vi "例4_IO.vi"() -> ()   [LabVIEW 2012]
panel:
  in  "EtherCAT  IO输出数":dbl
  in  "软件复位":bool
  in  "硬件复位":bool
  in  "总线状态":string
  in  "退出程序":bool
  in  "卡号":dbl
  in  "EtherCAT  IO输入数":dbl
  in  "15":bool
  in  "14":bool
  in  "7":bool
  in  "6":bool
  in  "13":bool
  in  "12":bool
  in  "11":bool
  in  "10":bool
  in  "9":bool
  in  "8":bool
  in  "5":bool
  in  "4":bool
  in  "3":bool
  in  "2":bool
  in  "1":bool
  in  "0":bool
  out "15":bool
  out "14":bool
  out "7":bool
  out "6":bool
  out "13":bool
  out "12":bool
  out "11":bool
  out "10":bool
  out "9":bool
  out "8":bool
  out "5":bool
  out "4":bool
  out "3":bool
  out "2":bool
  out "1":bool
  out "0":bool
  in  "7":bool
  in  "6":bool
  in  "5":bool
  in  "4":bool
  in  "3":bool
  in  "2":bool
  in  "1":bool
  in  "0":bool
  out "7":bool
  out "6":bool
  out "5":bool
  out "4":bool
  out "3":bool
  out "2":bool
  out "1":bool
  out "0":bool
  # "通用输入口（0~7）"
  # "EtherCAT  IO"
  # "通用输出口（0~7）"
  # "EtherCAT-输入口（0~15）"
  # "复位操作及总线状态"
  # "EtherCAT-输出口（0~15）"
  # "注：本例程位DMC—E3032总线卡接了一个EM32DX—E1EtherCAT总线IO扩展模块（16入16出）"
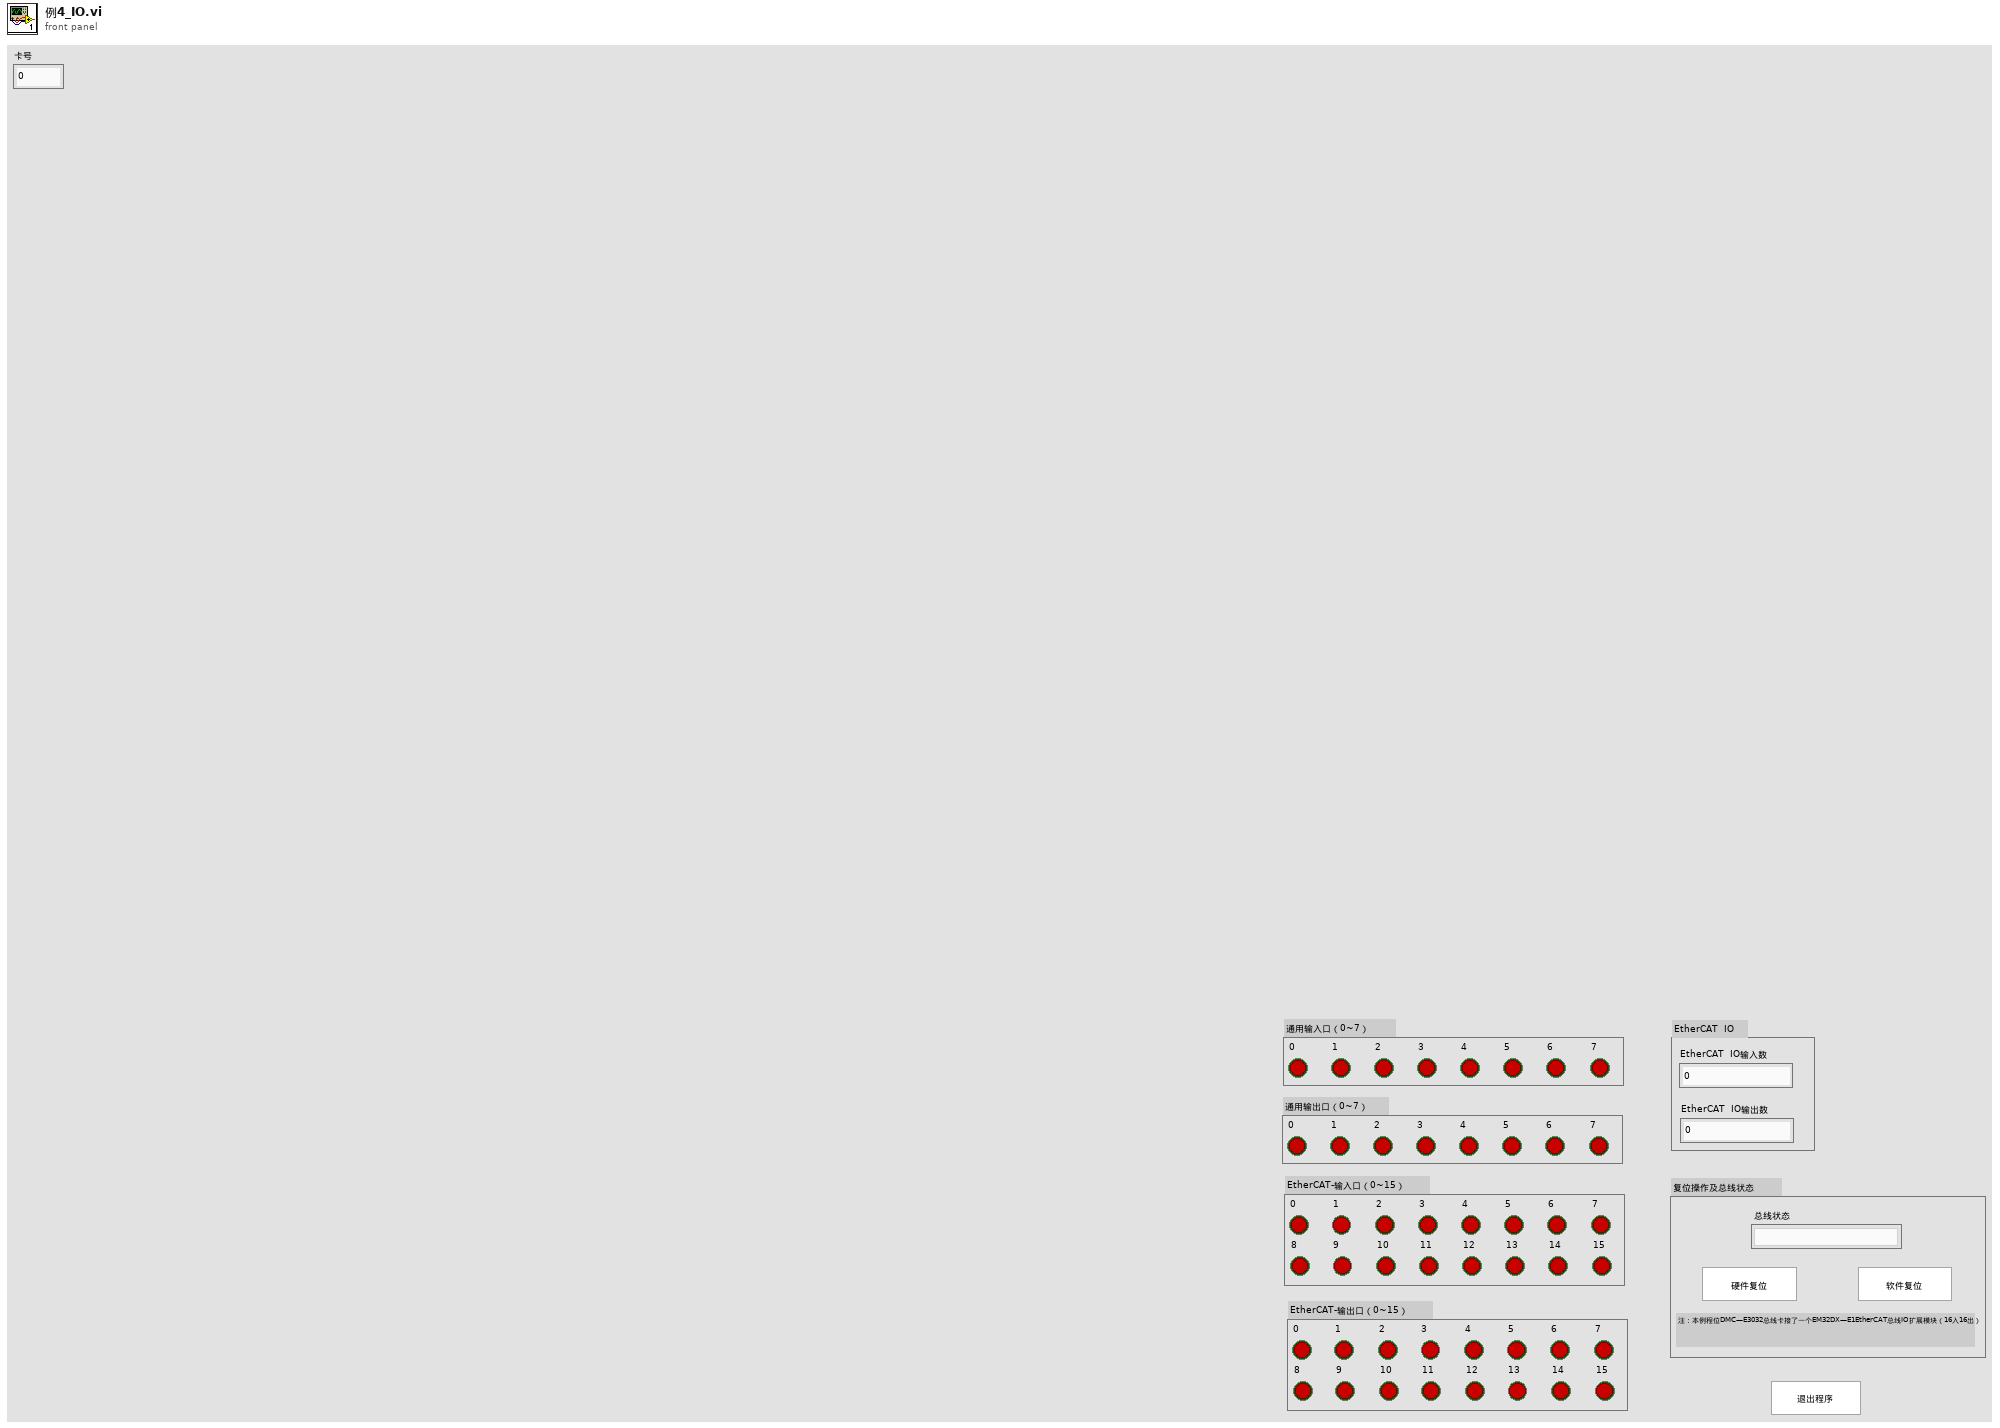
[diagram p1: front panel]
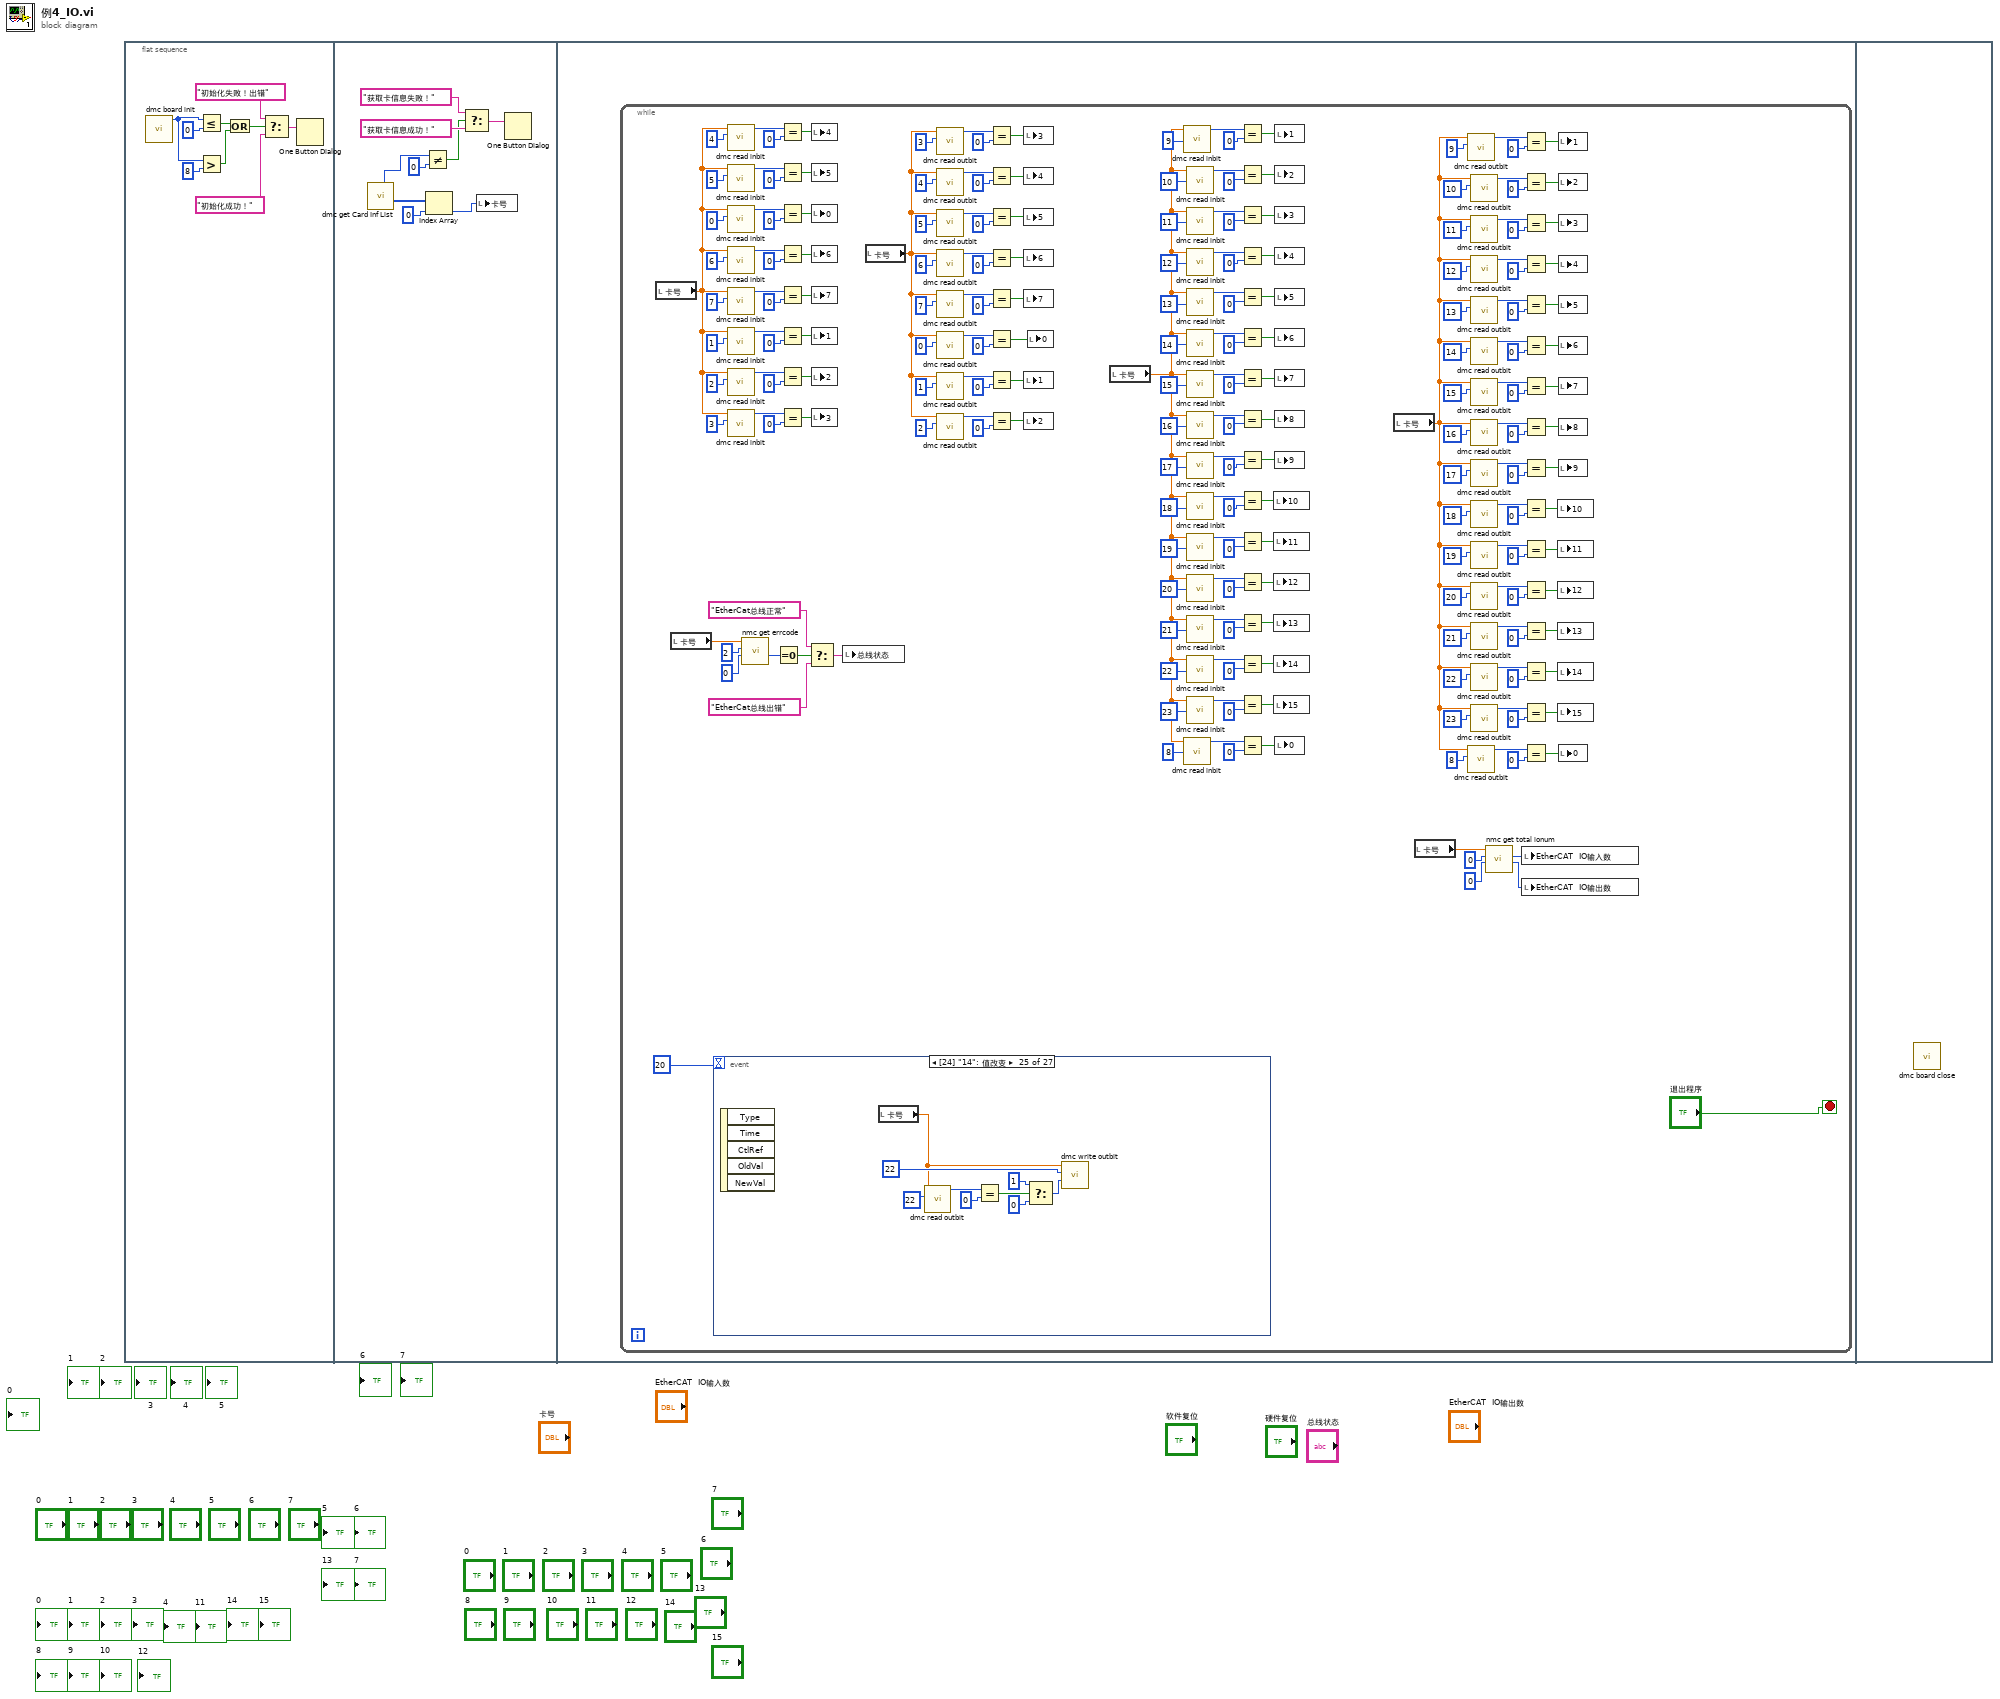
[diagram p0: block diagram]
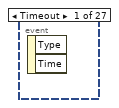
[diagram p2: hidden frame]
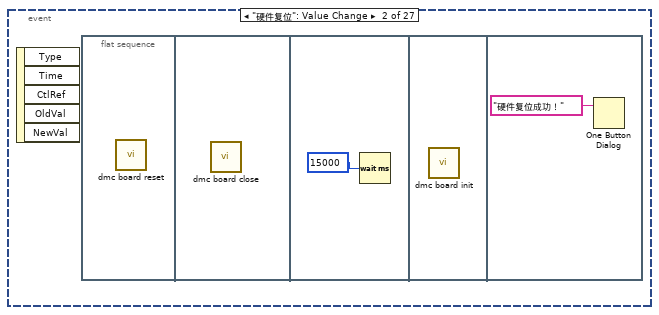
[diagram p3: hidden frame]
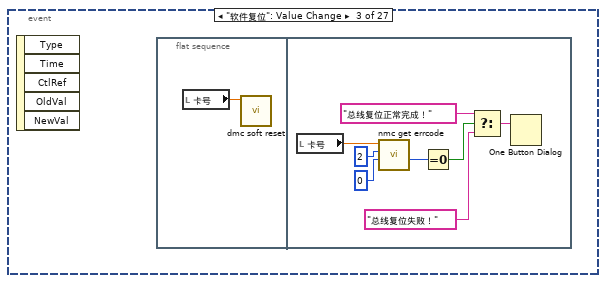
[diagram p4: hidden frame]
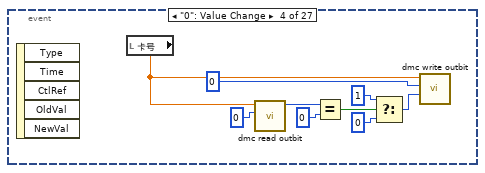
[diagram p5: hidden frame]
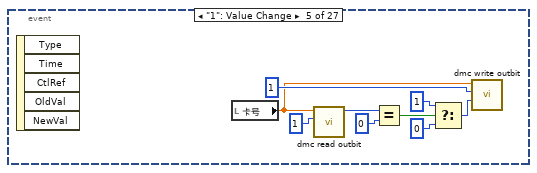
[diagram p6: hidden frame]
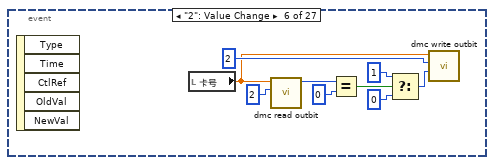
[diagram p7: hidden frame]
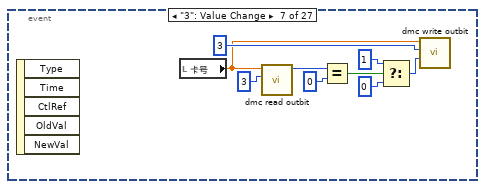
[diagram p8: hidden frame]
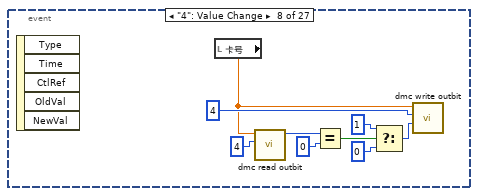
[diagram p9: hidden frame]
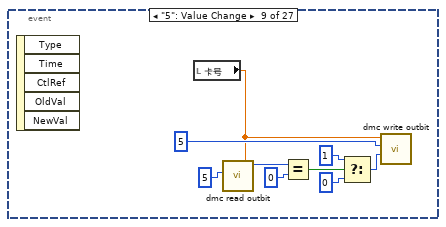
[diagram p10: hidden frame]
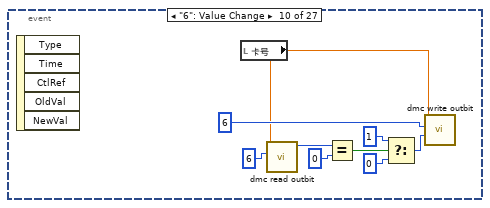
[diagram p11: hidden frame]
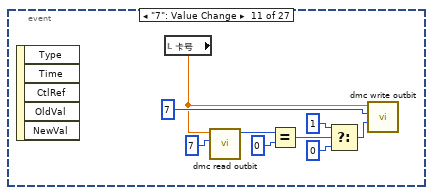
[diagram p12: hidden frame]
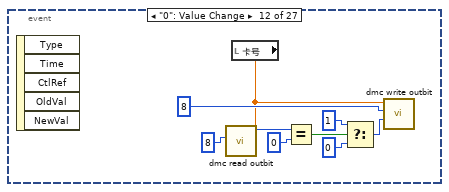
[diagram p13: hidden frame]
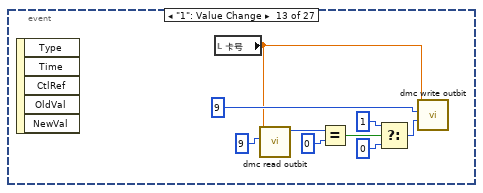
[diagram p14: hidden frame]
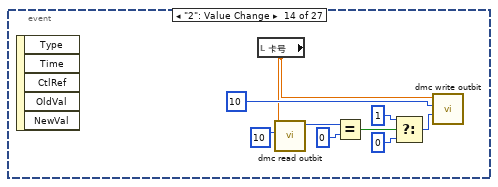
[diagram p15: hidden frame]
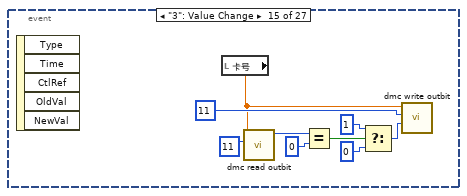
[diagram p16: hidden frame]
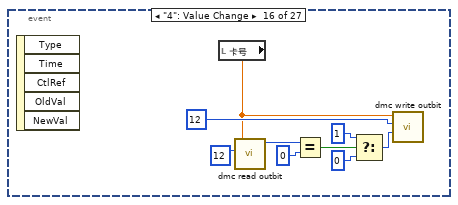
[diagram p17: hidden frame]
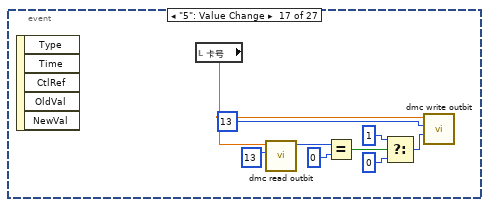
[diagram p18: hidden frame]
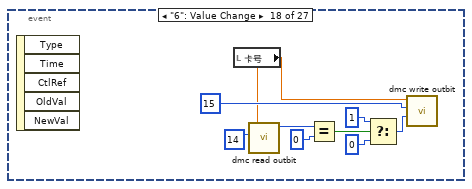
[diagram p19: hidden frame]
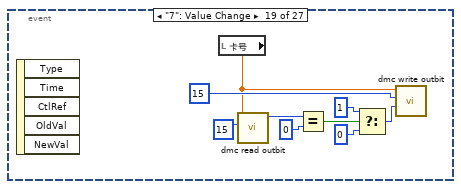
[diagram p20: hidden frame]
diagram:
  n1 = flat-sequence {
    frame #0 {
      n2 = call "dmc board init.vi"() -> ("function return"=w2:i16)  [unwired: 10 in, 1 out]
      n3 = Less Or Equal?(x=w2, y=0) -> (x <= y?=w5:bool)
      n4 = Greater?(x=w2, y=8) -> (0:w4:bool)
      n5 = Or(x=w5, y=w4) -> (x .or. y?=w6:bool)
      n6 = Select(t="初始化失败！出错", s=w6, f="初始化成功！") -> (s? t:f=w8:string)
      n7 = One Button Dialog(message=w8) -> ()  [unwired: 1 in, 1 out]
    }
    frame #1 {
      n8 = call "dmc get Card Inf List.vi"() -> ("CardIdList out"=w12:u16[], "function return"=w13:i16)  [unwired: 7 in, 3 out]
      n9 = Not Equal?(x=w13, y=0) -> (x != y?=w15:bool)
      n10 = Index Array(array=w12, index=0) -> (element=w10:u16)
      n11 = Select(t="获取卡信息失败！", s=w15, f="获取卡信息成功！") -> (s? t:f=w18:string)
      n12 = local write "卡号"(w10) -> ()
      n13 = One Button Dialog(message=w18) -> ()  [unwired: 1 in, 1 out]
    }
    frame #2 {
      n14 = while {
        stop <- "退出程序" stop-if-true
        n15 = local read "卡号"() -> (w197:dbl)
        n16 = local read "卡号"() -> (w19:dbl)
        n17 = event shown="[24] \"14\": 值改变" {
          selector: _ -> [_ _ _ _ _ _ _ _ _ _ _ _ _ _ _ _ _ _ _ _ _ _ _ _ _ _ _]
          dyn-events: _ -> [_ _ _ _ _ _ _ _ _ _ _ _ _ _ _ _ _ _ _ _ _ _ _ _ _ _ _]
          timeout: 20 -> [_ _ _ _ _ _ _ _ _ _ _ _ _ _ _ _ _ _ _ _ _ _ _ _ _ _ _]
          event Timeout {
            n18 = event-data() -> ()  [unwired: 1 in, 2 out]
          }
          event "硬件复位": Value Change {
            n19 = event-data() -> ()  [unwired: 1 in, 5 out]
            n20 = flat-sequence {
              frame #0 {
                n21 = call "dmc board reset.vi"() -> ()  [unwired: 10 in, 2 out]
              }
              frame #1 {
                n22 = call "dmc board close.vi"() -> ()  [unwired: 10 in, 2 out]
              }
              frame #2 {
                n23 = Wait (ms)(milliseconds to wait=15000) -> ()  [unwired: 1 out]
              }
              frame #3 {
                n24 = call "dmc board init.vi"() -> ()  [unwired: 10 in, 2 out]
              }
              frame #4 {
                n25 = One Button Dialog(message="硬件复位成功！") -> ()  [unwired: 1 in, 1 out]
              }
            }
          }
          event "软件复位": Value Change {
            n26 = event-data() -> ()  [unwired: 1 in, 5 out]
            n27 = flat-sequence {
              frame #0 {
                n28 = local read "卡号"() -> (w232:dbl)
                n29 = call "dmc soft reset.vi"("CardNo"=w232) -> ()  [unwired: 9 in, 2 out]
              }
              frame #1 {
                n30 = local read "卡号"() -> (w233:dbl)
                n31 = call "nmc get errcode.vi"("Errcode"=0, "channel"=2, "CardNo"=w233) -> ("Errcode out"=w237:u16)  [unwired: 6 in, 2 out]
                n32 = Equal To 0?(x=w237) -> (x = 0?=w238:bool)
                n33 = Select(t="总线复位正常完成！" ("当前状态"), s=w238, f="总线复位失败！" ("当前状态")) -> (s? t:f=w234:string)
                n34 = One Button Dialog(message=w234) -> ()  [unwired: 1 in, 1 out]
              }
            }
          }
          event "0": Value Change {
            n35 = event-data() -> ()  [unwired: 1 in, 5 out]
            n36 = local read "卡号"() -> (w241:dbl)
            n37 = call "dmc read outbit.vi"("bitno"=0, "CardNo"=w241) -> ("function return"=w248:i16)  [unwired: 8 in, 1 out]
            n38 = Equal?(x=w248, y=0) -> (x = y?=w246:bool)
            n39 = Select(t=1, s=w246, f=0) -> (s? t:f=w242:i32)
            n40 = call "dmc write outbit.vi"("on_off"=w242, "bitno"=0, "CardNo"=w241) -> ()  [unwired: 7 in, 2 out]
          }
          event "1": Value Change {
            n41 = event-data() -> ()  [unwired: 1 in, 5 out]
            n42 = local read "卡号"() -> (w250:dbl)
            n43 = call "dmc read outbit.vi"("bitno"=1, "CardNo"=w250) -> ("function return"=w257:i16)  [unwired: 8 in, 1 out]
            n44 = Equal?(x=w257, y=0) -> (x = y?=w255:bool)
            n45 = Select(t=1, s=w255, f=0) -> (s? t:f=w251:i32)
            n46 = call "dmc write outbit.vi"("on_off"=w251, "bitno"=1, "CardNo"=w250) -> ()  [unwired: 7 in, 2 out]
          }
          event "2": Value Change {
            n47 = event-data() -> ()  [unwired: 1 in, 5 out]
            n48 = local read "卡号"() -> (w259:dbl)
            n49 = call "dmc read outbit.vi"("bitno"=2, "CardNo"=w259) -> ("function return"=w266:i16)  [unwired: 8 in, 1 out]
            n50 = Equal?(x=w266, y=0) -> (x = y?=w264:bool)
            n51 = Select(t=1, s=w264, f=0) -> (s? t:f=w260:i32)
            n52 = call "dmc write outbit.vi"("on_off"=w260, "bitno"=2, "CardNo"=w259) -> ()  [unwired: 7 in, 2 out]
          }
          event "3": Value Change {
            n53 = event-data() -> ()  [unwired: 1 in, 5 out]
            n54 = local read "卡号"() -> (w268:dbl)
            n55 = call "dmc read outbit.vi"("bitno"=3, "CardNo"=w268) -> ("function return"=w275:i16)  [unwired: 8 in, 1 out]
            n56 = Equal?(x=w275, y=0) -> (x = y?=w273:bool)
            n57 = Select(t=1, s=w273, f=0) -> (s? t:f=w269:i32)
            n58 = call "dmc write outbit.vi"("on_off"=w269, "bitno"=3, "CardNo"=w268) -> ()  [unwired: 7 in, 2 out]
          }
          event "4": Value Change {
            n59 = event-data() -> ()  [unwired: 1 in, 5 out]
            n60 = local read "卡号"() -> (w277:dbl)
            n61 = call "dmc read outbit.vi"("bitno"=4, "CardNo"=w277) -> ("function return"=w284:i16)  [unwired: 8 in, 1 out]
            n62 = Equal?(x=w284, y=0) -> (x = y?=w282:bool)
            n63 = Select(t=1, s=w282, f=0) -> (s? t:f=w278:i32)
            n64 = call "dmc write outbit.vi"("on_off"=w278, "bitno"=4, "CardNo"=w277) -> ()  [unwired: 7 in, 2 out]
          }
          event "5": Value Change {
            n65 = event-data() -> ()  [unwired: 1 in, 5 out]
            n66 = local read "卡号"() -> (w286:dbl)
            n67 = call "dmc read outbit.vi"("bitno"=5, "CardNo"=w286) -> ("function return"=w288:i16)  [unwired: 8 in, 1 out]
            n68 = Equal?(x=w288, y=0) -> (x = y?=w290:bool)
            n69 = Select(t=1, s=w290, f=0) -> (s? t:f=w294:i32)
            n70 = call "dmc write outbit.vi"("on_off"=w294, "bitno"=5, "CardNo"=w286) -> ()  [unwired: 7 in, 2 out]
          }
          event "6": Value Change {
            n71 = event-data() -> ()  [unwired: 1 in, 5 out]
            n72 = local read "卡号"() -> (w295:dbl)
            n73 = call "dmc read outbit.vi"("bitno"=6, "CardNo"=w295) -> ("function return"=w302:i16)  [unwired: 8 in, 1 out]
            n74 = Equal?(x=w302, y=0) -> (x = y?=w300:bool)
            n75 = Select(t=1, s=w300, f=0) -> (s? t:f=w296:i32)
            n76 = call "dmc write outbit.vi"("on_off"=w296, "bitno"=6, "CardNo"=w295) -> ()  [unwired: 7 in, 2 out]
          }
          event "7": Value Change {
            n77 = event-data() -> ()  [unwired: 1 in, 5 out]
            n78 = local read "卡号"() -> (w304:dbl)
            n79 = call "dmc read outbit.vi"("bitno"=7, "CardNo"=w304) -> ("function return"=w311:i16)  [unwired: 8 in, 1 out]
            n80 = Equal?(x=w311, y=0) -> (x = y?=w309:bool)
            n81 = Select(t=1, s=w309, f=0) -> (s? t:f=w305:i32)
            n82 = call "dmc write outbit.vi"("on_off"=w305, "bitno"=7, "CardNo"=w304) -> ()  [unwired: 7 in, 2 out]
          }
          event "0": Value Change {
            n83 = event-data() -> ()  [unwired: 1 in, 5 out]
            n84 = local read "卡号"() -> (w313:dbl)
            n85 = call "dmc read outbit.vi"("bitno"=8, "CardNo"=w313) -> ("function return"=w320:i16)  [unwired: 8 in, 1 out]
            n86 = Equal?(x=w320, y=0) -> (x = y?=w318:bool)
            n87 = Select(t=1, s=w318, f=0) -> (s? t:f=w314:i32)
            n88 = call "dmc write outbit.vi"("on_off"=w314, "bitno"=8, "CardNo"=w313) -> ()  [unwired: 7 in, 2 out]
          }
          event "1": Value Change {
            n89 = event-data() -> ()  [unwired: 1 in, 5 out]
            n90 = local read "卡号"() -> (w322:dbl)
            n91 = call "dmc read outbit.vi"("bitno"=9, "CardNo"=w322) -> ("function return"=w329:i16)  [unwired: 8 in, 1 out]
            n92 = Equal?(x=w329, y=0) -> (x = y?=w327:bool)
            n93 = Select(t=1, s=w327, f=0) -> (s? t:f=w323:i32)
            n94 = call "dmc write outbit.vi"("on_off"=w323, "bitno"=9, "CardNo"=w322) -> ()  [unwired: 7 in, 2 out]
          }
          event "2": Value Change {
            n95 = event-data() -> ()  [unwired: 1 in, 5 out]
            n96 = local read "卡号"() -> (w331:dbl)
            n97 = call "dmc read outbit.vi"("bitno"=10, "CardNo"=w331) -> ("function return"=w338:i16)  [unwired: 8 in, 1 out]
            n98 = Equal?(x=w338, y=0) -> (x = y?=w336:bool)
            n99 = Select(t=1, s=w336, f=0) -> (s? t:f=w332:i32)
            n100 = call "dmc write outbit.vi"("on_off"=w332, "bitno"=10, "CardNo"=w331) -> ()  [unwired: 7 in, 2 out]
          }
          event "3": Value Change {
            n101 = event-data() -> ()  [unwired: 1 in, 5 out]
            n102 = local read "卡号"() -> (w340:dbl)
            n103 = call "dmc read outbit.vi"("bitno"=11, "CardNo"=w340) -> ("function return"=w347:i16)  [unwired: 8 in, 1 out]
            n104 = Equal?(x=w347, y=0) -> (x = y?=w345:bool)
            n105 = Select(t=1, s=w345, f=0) -> (s? t:f=w341:i32)
            n106 = call "dmc write outbit.vi"("on_off"=w341, "bitno"=11, "CardNo"=w340) -> ()  [unwired: 7 in, 2 out]
          }
          event "4": Value Change {
            n107 = event-data() -> ()  [unwired: 1 in, 5 out]
            n108 = local read "卡号"() -> (w349:dbl)
            n109 = call "dmc read outbit.vi"("bitno"=12, "CardNo"=w349) -> ("function return"=w356:i16)  [unwired: 8 in, 1 out]
            n110 = Equal?(x=w356, y=0) -> (x = y?=w354:bool)
            n111 = Select(t=1, s=w354, f=0) -> (s? t:f=w350:i32)
            n112 = call "dmc write outbit.vi"("on_off"=w350, "bitno"=12, "CardNo"=w349) -> ()  [unwired: 7 in, 2 out]
          }
          event "5": Value Change {
            n113 = event-data() -> ()  [unwired: 1 in, 5 out]
            n114 = local read "卡号"() -> (w358:dbl)
            n115 = call "dmc read outbit.vi"("bitno"=13, "CardNo"=w358) -> ("function return"=w360:i16)  [unwired: 8 in, 1 out]
            n116 = Equal?(x=w360, y=0) -> (x = y?=w362:bool)
            n117 = Select(t=1, s=w362, f=0) -> (s? t:f=w366:i32)
            n118 = call "dmc write outbit.vi"("on_off"=w366, "bitno"=13, "CardNo"=w358) -> ()  [unwired: 7 in, 2 out]
          }
          event "6": Value Change {
            n119 = event-data() -> ()  [unwired: 1 in, 5 out]
            n120 = local read "卡号"() -> (w367:dbl)
            n121 = call "dmc read outbit.vi"("bitno"=14, "CardNo"=w367) -> ("function return"=w374:i16)  [unwired: 8 in, 1 out]
            n122 = Equal?(x=w374, y=0) -> (x = y?=w372:bool)
            n123 = Select(t=1, s=w372, f=0) -> (s? t:f=w368:i32)
            n124 = call "dmc write outbit.vi"("on_off"=w368, "bitno"=15, "CardNo"=w367) -> ()  [unwired: 7 in, 2 out]
          }
          event "7": Value Change {
            n125 = event-data() -> ()  [unwired: 1 in, 5 out]
            n126 = local read "卡号"() -> (w376:dbl)
            n127 = call "dmc read outbit.vi"("bitno"=15, "CardNo"=w376) -> ("function return"=w383:i16)  [unwired: 8 in, 1 out]
            n128 = Equal?(x=w383, y=0) -> (x = y?=w381:bool)
            n129 = Select(t=1, s=w381, f=0) -> (s? t:f=w377:i32)
            n130 = call "dmc write outbit.vi"("on_off"=w377, "bitno"=15, "CardNo"=w376) -> ()  [unwired: 7 in, 2 out]
          }
          event "8": Value Change {
            n131 = event-data() -> ()  [unwired: 1 in, 5 out]
            n132 = local read "卡号"() -> (w385:dbl)
            n133 = call "dmc read outbit.vi"("bitno"=16, "CardNo"=w385) -> ("function return"=w392:i16)  [unwired: 8 in, 1 out]
            n134 = Equal?(x=w392, y=0) -> (x = y?=w390:bool)
            n135 = Select(t=1, s=w390, f=0) -> (s? t:f=w386:i32)
            n136 = call "dmc write outbit.vi"("on_off"=w386, "bitno"=16, "CardNo"=w385) -> ()  [unwired: 7 in, 2 out]
          }
          event "9": Value Change {
            n137 = event-data() -> ()  [unwired: 1 in, 5 out]
            n138 = local read "卡号"() -> (w394:dbl)
            n139 = call "dmc read outbit.vi"("bitno"=17, "CardNo"=w394) -> ("function return"=w396:i16)  [unwired: 8 in, 1 out]
            n140 = Equal?(x=w396, y=0) -> (x = y?=w398:bool)
            n141 = Select(t=1, s=w398, f=0) -> (s? t:f=w402:i32)
            n142 = call "dmc write outbit.vi"("on_off"=w402, "bitno"=17, "CardNo"=w394) -> ()  [unwired: 7 in, 2 out]
          }
          event "10": Value Change {
            n143 = event-data() -> ()  [unwired: 1 in, 5 out]
            n144 = local read "卡号"() -> (w403:dbl)
            n145 = call "dmc read outbit.vi"("bitno"=18, "CardNo"=w403) -> ("function return"=w410:i16)  [unwired: 8 in, 1 out]
            n146 = Equal?(x=w410, y=0) -> (x = y?=w408:bool)
            n147 = Select(t=1, s=w408, f=0) -> (s? t:f=w404:i32)
            n148 = call "dmc write outbit.vi"("on_off"=w404, "bitno"=18, "CardNo"=w403) -> ()  [unwired: 7 in, 2 out]
          }
          event "12": Value Change {
            n149 = event-data() -> ()  [unwired: 1 in, 5 out]
            n150 = local read "卡号"() -> (w412:dbl)
            n151 = call "dmc read outbit.vi"("bitno"=20, "CardNo"=w412) -> ("function return"=w419:i16)  [unwired: 8 in, 1 out]
            n152 = Equal?(x=w419, y=0) -> (x = y?=w417:bool)
            n153 = Select(t=1, s=w417, f=0) -> (s? t:f=w413:i32)
            n154 = call "dmc write outbit.vi"("on_off"=w413, "bitno"=20, "CardNo"=w412) -> ()  [unwired: 7 in, 2 out]
          }
          event "13": Value Change {
            n155 = event-data() -> ()  [unwired: 1 in, 5 out]
            n156 = local read "卡号"() -> (w421:dbl)
            n157 = call "dmc read outbit.vi"("bitno"=21, "CardNo"=w421) -> ("function return"=w428:i16)  [unwired: 8 in, 1 out]
            n158 = Equal?(x=w428, y=0) -> (x = y?=w426:bool)
            n159 = Select(t=1, s=w426, f=0) -> (s? t:f=w422:i32)
            n160 = call "dmc write outbit.vi"("on_off"=w422, "bitno"=21, "CardNo"=w421) -> ()  [unwired: 7 in, 2 out]
          }
          event "14": Value Change {
            n161 = event-data() -> ()  [unwired: 1 in, 5 out]
            n162 = local read "卡号"() -> (w430:dbl)
            n163 = call "dmc read outbit.vi"("bitno"=22, "CardNo"=w430) -> ("function return"=w437:i16)  [unwired: 8 in, 1 out]
            n164 = Equal?(x=w437, y=0) -> (x = y?=w435:bool)
            n165 = Select(t=1, s=w435, f=0) -> (s? t:f=w431:i32)
            n166 = call "dmc write outbit.vi"("on_off"=w431, "bitno"=22, "CardNo"=w430) -> ()  [unwired: 7 in, 2 out]
          }
          event "15": Value Change {
            n167 = event-data() -> ()  [unwired: 1 in, 5 out]
            n168 = local read "卡号"() -> (w439:dbl)
            n169 = call "dmc read outbit.vi"("bitno"=23, "CardNo"=w439) -> ("function return"=w446:i16)  [unwired: 8 in, 1 out]
            n170 = Equal?(x=w446, y=0) -> (x = y?=w444:bool)
            n171 = Select(t=1, s=w444, f=0) -> (s? t:f=w440:i32)
            n172 = call "dmc write outbit.vi"("on_off"=w440, "bitno"=23, "CardNo"=w439) -> ()  [unwired: 7 in, 2 out]
          }
          event "11": Value Change {
            n173 = event-data() -> ()  [unwired: 1 in, 5 out]
            n174 = local read "卡号"() -> (w448:dbl)
            n175 = call "dmc read outbit.vi"("bitno"=19, "CardNo"=w448) -> ("function return"=w455:i16)  [unwired: 8 in, 1 out]
            n176 = Equal?(x=w455, y=0) -> (x = y?=w453:bool)
            n177 = Select(t=1, s=w453, f=0) -> (s? t:f=w449:i32)
            n178 = call "dmc write outbit.vi"("on_off"=w449, "bitno"=19, "CardNo"=w448) -> ()  [unwired: 7 in, 2 out]
          }
        }
        n179 = call "dmc read inbit.vi"("bitno"=4, "CardNo"=w197) -> ("function return"=w211:i16)  [unwired: 8 in, 1 out]
        n180 = call "dmc read inbit.vi"("bitno"=5, "CardNo"=w197) -> ("function return"=w207:i16)  [unwired: 8 in, 1 out]
        n181 = call "dmc read inbit.vi"("bitno"=0, "CardNo"=w197) -> ("function return"=w228:i16)  [unwired: 8 in, 1 out]
        n182 = call "dmc read inbit.vi"("bitno"=6, "CardNo"=w197) -> ("function return"=w203:i16)  [unwired: 8 in, 1 out]
        n183 = call "dmc read inbit.vi"("bitno"=7, "CardNo"=w197) -> ("function return"=w200:i16)  [unwired: 8 in, 1 out]
        n184 = call "dmc read inbit.vi"("bitno"=1, "CardNo"=w197) -> ("function return"=w222:i16)  [unwired: 8 in, 1 out]
        n185 = call "dmc read inbit.vi"("bitno"=2, "CardNo"=w197) -> ("function return"=w218:i16)  [unwired: 8 in, 1 out]
        n186 = call "dmc read inbit.vi"("bitno"=3, "CardNo"=w197) -> ("function return"=w215:i16)  [unwired: 8 in, 1 out]
        n187 = call "nmc get errcode.vi"("Errcode"=0, "channel"=2, "CardNo"=w19) -> ("Errcode out"=w24:u16)  [unwired: 6 in, 2 out]
        n188 = Equal To 0?(x=w24) -> (x = 0?=w23:bool)
        n189 = Equal?(x=w211, y=0) -> (x = y?=w210:bool)
        n190 = Equal?(x=w207, y=0) -> (x = y?=w206:bool)
        n191 = Equal?(x=w228, y=0) -> (x = y?=w226:bool)
        n192 = Equal?(x=w203, y=0) -> (x = y?=w202:bool)
        n193 = Equal?(x=w200, y=0) -> (x = y?=w199:bool)
        n194 = Equal?(x=w222, y=0) -> (x = y?=w223:bool)
        n195 = Equal?(x=w218, y=0) -> (x = y?=w219:bool)
        n196 = Equal?(x=w215, y=0) -> (x = y?=w214:bool)
        n197 = Select(t="EtherCat总线正常" ("当前状态"), s=w23, f="EtherCat总线出错" ("当前状态")) -> (s? t:f=w20:string)
        n198 = local write "4"(w210) -> ()
        n199 = local write "5"(w206) -> ()
        n200 = local write "0"(w226) -> ()
        n201 = local write "6"(w202) -> ()
        n202 = local write "7"(w199) -> ()
        n203 = local write "1"(w223) -> ()
        n204 = local write "2"(w219) -> ()
        n205 = local write "3"(w214) -> ()
        n206 = local write "总线状态"(w20) -> ()
        n207 = local read "卡号"() -> (w164:dbl)
        n208 = call "dmc read outbit.vi"("bitno"=3, "CardNo"=w164) -> ("function return"=w184:i16)  [unwired: 8 in, 1 out]
        n209 = call "dmc read outbit.vi"("bitno"=4, "CardNo"=w164) -> ("function return"=w181:i16)  [unwired: 8 in, 1 out]
        n210 = call "dmc read outbit.vi"("bitno"=5, "CardNo"=w164) -> ("function return"=w178:i16)  [unwired: 8 in, 1 out]
        n211 = call "dmc read outbit.vi"("bitno"=6, "CardNo"=w164) -> ("function return"=w175:i16)  [unwired: 8 in, 1 out]
        n212 = call "dmc read outbit.vi"("bitno"=7, "CardNo"=w164) -> ("function return"=w172:i16)  [unwired: 8 in, 1 out]
        n213 = call "dmc read outbit.vi"("bitno"=0, "CardNo"=w164) -> ("function return"=w194:i16)  [unwired: 8 in, 1 out]
        n214 = call "dmc read outbit.vi"("bitno"=1, "CardNo"=w164) -> ("function return"=w190:i16)  [unwired: 8 in, 1 out]
        n215 = call "dmc read outbit.vi"("bitno"=2, "CardNo"=w164) -> ("function return"=w187:i16)  [unwired: 8 in, 1 out]
        n216 = Equal?(x=w184, y=0) -> (x = y?=w166:bool)
        n217 = Equal?(x=w181, y=0) -> (x = y?=w167:bool)
        n218 = Equal?(x=w178, y=0) -> (x = y?=w168:bool)
        n219 = Equal?(x=w175, y=0) -> (x = y?=w169:bool)
        n220 = Equal?(x=w172, y=0) -> (x = y?=w170:bool)
        n221 = Equal?(x=w194, y=0) -> (x = y?=w193:bool)
        n222 = Equal?(x=w190, y=0) -> (x = y?=w171:bool)
        n223 = Equal?(x=w187, y=0) -> (x = y?=w165:bool)
        n224 = local write "3"(w166) -> ()
        n225 = local write "4"(w167) -> ()
        n226 = local write "5"(w168) -> ()
        n227 = local write "6"(w169) -> ()
        n228 = local write "7"(w170) -> ()
        n229 = local write "1"(w171) -> ()
        n230 = local write "2"(w165) -> ()
        n231 = local write "0"(w193) -> ()
        n232 = local read "卡号"() -> (w115:dbl)
        n233 = call "dmc read inbit.vi"("bitno"=9, "CardNo"=w115) -> ("function return"=w157:i16)  [unwired: 8 in, 1 out]
        n234 = call "dmc read inbit.vi"("bitno"=8, "CardNo"=w115) -> ("function return"=w158:i16)  [unwired: 8 in, 1 out]
        n235 = call "dmc read inbit.vi"("bitno"=10, "CardNo"=w115) -> ("function return"=w161:i16)  [unwired: 8 in, 1 out]
        n236 = call "dmc read inbit.vi"("bitno"=11, "CardNo"=w115) -> ("function return"=w156:i16)  [unwired: 8 in, 1 out]
        n237 = call "dmc read inbit.vi"("bitno"=12, "CardNo"=w115) -> ("function return"=w155:i16)  [unwired: 8 in, 1 out]
        n238 = call "dmc read inbit.vi"("bitno"=13, "CardNo"=w115) -> ("function return"=w160:i16)  [unwired: 8 in, 1 out]
        n239 = call "dmc read inbit.vi"("bitno"=14, "CardNo"=w115) -> ("function return"=w109:i16)  [unwired: 8 in, 1 out]
        n240 = call "dmc read inbit.vi"("bitno"=15, "CardNo"=w115) -> ("function return"=w159:i16)  [unwired: 8 in, 1 out]
        n241 = call "dmc read inbit.vi"("bitno"=16, "CardNo"=w115) -> ("function return"=w151:i16)  [unwired: 8 in, 1 out]
        n242 = call "dmc read inbit.vi"("bitno"=17, "CardNo"=w115) -> ("function return"=w150:i16)  [unwired: 8 in, 1 out]
        n243 = call "dmc read inbit.vi"("bitno"=18, "CardNo"=w115) -> ("function return"=w114:i16)  [unwired: 8 in, 1 out]
        n244 = call "dmc read inbit.vi"("bitno"=19, "CardNo"=w115) -> ("function return"=w149:i16)  [unwired: 8 in, 1 out]
        n245 = call "dmc read inbit.vi"("bitno"=20, "CardNo"=w115) -> ("function return"=w148:i16)  [unwired: 8 in, 1 out]
        n246 = call "dmc read inbit.vi"("bitno"=21, "CardNo"=w115) -> ("function return"=w154:i16)  [unwired: 8 in, 1 out]
        n247 = call "dmc read inbit.vi"("bitno"=22, "CardNo"=w115) -> ("function return"=w153:i16)  [unwired: 8 in, 1 out]
        n248 = call "dmc read inbit.vi"("bitno"=23, "CardNo"=w115) -> ("function return"=w152:i16)  [unwired: 8 in, 1 out]
        n249 = Equal?(x=w157, y=0) -> (x = y?=w130:bool)
        n250 = Equal?(x=w161, y=0) -> (x = y?=w129:bool)
        n251 = Equal?(x=w156, y=0) -> (x = y?=w128:bool)
        n252 = Equal?(x=w155, y=0) -> (x = y?=w127:bool)
        n253 = Equal?(x=w160, y=0) -> (x = y?=w126:bool)
        n254 = Equal?(x=w109, y=0) -> (x = y?=w125:bool)
        n255 = Equal?(x=w159, y=0) -> (x = y?=w124:bool)
        n256 = Equal?(x=w151, y=0) -> (x = y?=w123:bool)
        n257 = Equal?(x=w150, y=0) -> (x = y?=w122:bool)
        n258 = Equal?(x=w114, y=0) -> (x = y?=w121:bool)
        n259 = Equal?(x=w149, y=0) -> (x = y?=w120:bool)
        n260 = Equal?(x=w148, y=0) -> (x = y?=w119:bool)
        n261 = Equal?(x=w154, y=0) -> (x = y?=w118:bool)
        n262 = Equal?(x=w153, y=0) -> (x = y?=w117:bool)
        n263 = Equal?(x=w152, y=0) -> (x = y?=w116:bool)
        n264 = Equal?(x=w158, y=0) -> (x = y?=w131:bool)
        n265 = local write "10"(w121) -> ()
        n266 = local write "11"(w120) -> ()
        n267 = local write "12"(w119) -> ()
        n268 = local write "13"(w118) -> ()
        n269 = local write "14"(w117) -> ()
        n270 = local write "15"(w116) -> ()
        n271 = local write "1"(w130) -> ()
        n272 = local write "2"(w129) -> ()
        n273 = local write "3"(w128) -> ()
        n274 = local write "4"(w127) -> ()
        n275 = local write "5"(w126) -> ()
        n276 = local write "6"(w125) -> ()
        n277 = local write "7"(w124) -> ()
        n278 = local write "8"(w123) -> ()
        n279 = local write "9"(w122) -> ()
        n280 = local write "0"(w131) -> ()
        n281 = local read "卡号"() -> (w48:dbl)
        n282 = local read "卡号"() -> (w31:dbl)
        n283 = call "dmc read outbit.vi"("bitno"=9, "CardNo"=w48) -> ("function return"=w89:i16)  [unwired: 8 in, 1 out]
        n284 = call "dmc read outbit.vi"("bitno"=8, "CardNo"=w48) -> ("function return"=w91:i16)  [unwired: 8 in, 1 out]
        n285 = call "dmc read outbit.vi"("bitno"=10, "CardNo"=w48) -> ("function return"=w87:i16)  [unwired: 8 in, 1 out]
        n286 = call "dmc read outbit.vi"("bitno"=11, "CardNo"=w48) -> ("function return"=w85:i16)  [unwired: 8 in, 1 out]
        n287 = call "dmc read outbit.vi"("bitno"=12, "CardNo"=w48) -> ("function return"=w83:i16)  [unwired: 8 in, 1 out]
        n288 = call "dmc read outbit.vi"("bitno"=13, "CardNo"=w48) -> ("function return"=w97:i16)  [unwired: 8 in, 1 out]
        n289 = call "dmc read outbit.vi"("bitno"=14, "CardNo"=w48) -> ("function return"=w95:i16)  [unwired: 8 in, 1 out]
        n290 = call "dmc read outbit.vi"("bitno"=15, "CardNo"=w48) -> ("function return"=w93:i16)  [unwired: 8 in, 1 out]
        n291 = call "dmc read outbit.vi"("bitno"=16, "CardNo"=w48) -> ("function return"=w75:i16)  [unwired: 8 in, 1 out]
        n292 = call "dmc read outbit.vi"("bitno"=17, "CardNo"=w48) -> ("function return"=w73:i16)  [unwired: 8 in, 1 out]
        n293 = call "dmc read outbit.vi"("bitno"=18, "CardNo"=w48) -> ("function return"=w71:i16)  [unwired: 8 in, 1 out]
        n294 = call "dmc read outbit.vi"("bitno"=19, "CardNo"=w48) -> ("function return"=w69:i16)  [unwired: 8 in, 1 out]
        n295 = call "dmc read outbit.vi"("bitno"=20, "CardNo"=w48) -> ("function return"=w67:i16)  [unwired: 8 in, 1 out]
        n296 = call "dmc read outbit.vi"("bitno"=21, "CardNo"=w48) -> ("function return"=w81:i16)  [unwired: 8 in, 1 out]
        n297 = call "dmc read outbit.vi"("bitno"=22, "CardNo"=w48) -> ("function return"=w79:i16)  [unwired: 8 in, 1 out]
        n298 = call "dmc read outbit.vi"("bitno"=23, "CardNo"=w48) -> ("function return"=w77:i16)  [unwired: 8 in, 1 out]
        n299 = call "nmc get total ionum.vi"("TotalOut"=0, "TotalIn"=0, "CardNo"=w31) -> ("TotalOut out"=w27:u16, "TotalIn out"=w28:u16)  [unwired: 5 in, 2 out]
        n300 = local write "EtherCAT  IO输入数"(w28) -> ()
        n301 = local write "EtherCAT  IO输出数"(w27) -> ()
        n302 = Equal?(x=w89, y=0) -> (x = y?=w46:bool)
        n303 = Equal?(x=w87, y=0) -> (x = y?=w45:bool)
        n304 = Equal?(x=w85, y=0) -> (x = y?=w44:bool)
        n305 = Equal?(x=w83, y=0) -> (x = y?=w43:bool)
        n306 = Equal?(x=w97, y=0) -> (x = y?=w42:bool)
        n307 = Equal?(x=w95, y=0) -> (x = y?=w41:bool)
        n308 = Equal?(x=w93, y=0) -> (x = y?=w40:bool)
        n309 = Equal?(x=w75, y=0) -> (x = y?=w39:bool)
        n310 = Equal?(x=w73, y=0) -> (x = y?=w38:bool)
        n311 = Equal?(x=w71, y=0) -> (x = y?=w37:bool)
        n312 = Equal?(x=w69, y=0) -> (x = y?=w36:bool)
        n313 = Equal?(x=w67, y=0) -> (x = y?=w35:bool)
        n314 = Equal?(x=w81, y=0) -> (x = y?=w34:bool)
        n315 = Equal?(x=w79, y=0) -> (x = y?=w33:bool)
        n316 = Equal?(x=w77, y=0) -> (x = y?=w32:bool)
        n317 = Equal?(x=w91, y=0) -> (x = y?=w47:bool)
        n318 = local write "10"(w37) -> ()
        n319 = local write "11"(w36) -> ()
        n320 = local write "12"(w35) -> ()
        n321 = local write "13"(w34) -> ()
        n322 = local write "14"(w33) -> ()
        n323 = local write "15"(w32) -> ()
        n324 = local write "1"(w46) -> ()
        n325 = local write "2"(w45) -> ()
        n326 = local write "3"(w44) -> ()
        n327 = local write "4"(w43) -> ()
        n328 = local write "5"(w42) -> ()
        n329 = local write "6"(w41) -> ()
        n330 = local write "7"(w40) -> ()
        n331 = local write "8"(w39) -> ()
        n332 = local write "9"(w38) -> ()
        n333 = local write "0"(w47) -> ()
      }
    }
    frame #3 {
      n334 = call "dmc board close.vi"() -> ()  [unwired: 10 in, 2 out]
    }
  }
